vi "peg_leg_state_store.vi"(10 "data_store_mode":enum16{"Set", "Get"}(ring), 11 "peg_leg_state":T1=enum."down") -> (2 "Initialized":bool, 3 "peg_leg_state out":T1=enum."down")   [LabVIEW 2011]
uses:
  peg_leg_state.ctl
  <vilib>/Rock Robotics/WPI/DriverStation/WPI_DriverStationCommDataCacheOp.ctl
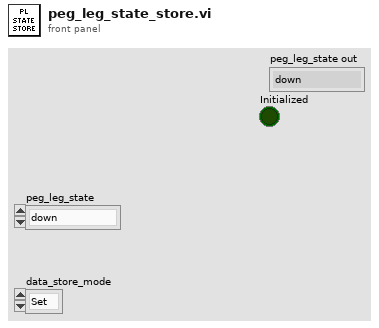
[diagram p1: front panel]
types:
  T1 = typedef "peg_leg_state.ctl" = enum16{"up", "down", "unfold", "manual"}
  T2 = typedef "WPI_DriverStationCommDataCacheOp.ctl" = enum16{"Get", "Set", "Init"}
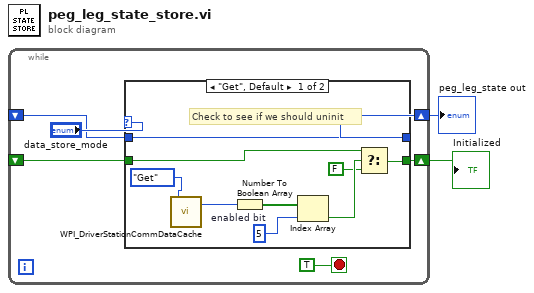
[diagram p0: block diagram]
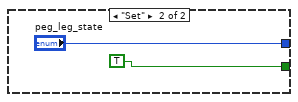
[diagram p2: hidden frame]
diagram:
  n1 = while {
    shift-right: [w6] -> w2
    shift-left: _ -> [w5]
    shift-right: [w4] -> w1
    shift-left: _ -> [w3]
    stop <- TRUE stop-if-true
    n2 = case shown="\"Get\", Default" "data_store_mode" {
      tunnel: [w17 "peg_leg_state"] -> w6
      tunnel: w5 -> [w17 _]
      tunnel: [w10 TRUE] -> w4
      tunnel: w3 -> [w11 _]
      frame "Get", Default {
        w15 = 5  # enabled bit
        # "Check to see if we should uninit"
        n3 = call <vilib>:"WPI_DriverStationCommDataCache.vi"("CommDataCacheOp"=WPI_DriverStationCommDataCacheOp."Get") -> ("ControlBit out"=w13:u8)  [unwired: 18 out]
        n4 = Number To Boolean Array(number=w13) -> (Boolean array=w14:bool[])
        n5 = Index Array(array=w14, index=w15) -> (element=w12:bool)
        n6 = Select(t=w11, s=w12, f=FALSE) -> (s? t:f=w10:bool)
      }
      frame "Set" {
      }
    }
  }
  "peg_leg_state out" <- w2
  "Initialized" <- w1
